vi "PH_Beckhoff.scale digital Beckhoff Value.vi"(0 "Beckhoff value":bool, 1 "inverted?":bool) -> (2 "DIM value":bool)   [LabVIEW 2014, in "PH_Beckhoff.lvlib"]
doc: "This VI is forseen to scale (this means: invert) the raw digital Beckhoff value to the DIM value to be published."
uses:
  PH_Beckhoff.lvlib
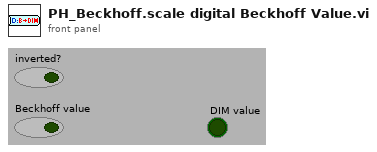
[diagram p1: front panel]
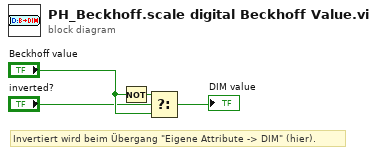
[diagram p0: block diagram]
diagram:
  # "Invertiert wird beim Übergang \"Eigene Attribute -> DIM\" (hier)."
  n1 = Not(x="Beckhoff value") -> (.not. x?=w3:bool)
  n2 = Select(t=w3, s="inverted?", f="Beckhoff value") -> (s? t:f=→"DIM value":bool)
